vi "Read Aout Span.vi"(8 "error in (no error)":errorcluster, 11 "VISA resource name":refnum<visa-resource-name>) -> (0 "error out":errorcluster, 2 "aout span":cluster{"ASpanC":dbl, "ASpanL":dbl}={"ASpanC"=20.0, "ASpanL"=20.0}, 3 "VISA resource name out":refnum<visa-resource-name>)   [LabVIEW 2019, in "Andeen-Hagerling 2700A.lvlib"]
doc: "Returns the analog out span parameter.\n\nAnalog out span is the the distance between the upper and lower analog output\nvoltage bounds for capacitance and/or loss in volts. These\nanalog output voltage spans correspond directly to the input\ndeviation capacitance and loss spans."
uses:
  Andeen-Hagerling 2700A.lvlib
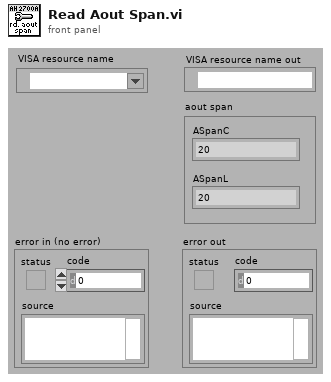
[diagram p1: front panel]
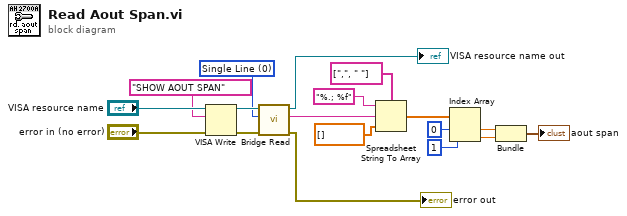
[diagram p0: block diagram]
diagram:
  w1 = u16 0 items=["Single Line", "Multi-Line"] ("Multiline")
  n1 = VISA Write(VISA resource name="VISA resource name", write buffer="SHOW AOUT SPAN" ("command"), error in (no error)="error in (no error)") -> (VISA resource name out=w16:refnum<visa-resource-name>, error out=w15:errorcluster)  [unwired: 1 out]
  n2 = call "Bridge Read.vi"("error in (no error)"=w15, "multiline"=w1, "VISA resource name"=w16) -> ("error out"=→"error out":errorcluster, "read buffer"=w10:string, "VISA resource name out"=→"VISA resource name out":refnum<visa-resource-name>)  [unwired: 6 in]
  n3 = Spreadsheet String To Array(delimiter (Tab)=string[] [",", " "], format string="%.; %f", spreadsheet string=w10, array type (2D Dbl)=dbl[] []) -> (array=w5:dbl[])
  n4 = Index Array(array=w5, index #1=0 ("index"), index #2=1 ("index")) -> (element #1=w4:dbl, element #2=w3:dbl)
  n5 = Bundle(w4, w3) -> (→"aout span":cluster{dbl, dbl})  [unwired: 1 in]
